vi "User.LoginGui.vi"(11 "Try only (T)":bool=TRUE) -> (2 "UserLevelOut":T1 caption="User Level Out", 3 "ok?":bool)   [LabVIEW 2013]
uses:
  User.LoginGui.Action.ctl
  User.Global.vi
  User.Level.ctl
  Config/Config.Global.vi
panel:
  out "_loop":i32(ring)=4
  in  "open?":bool
  out "_GuruPeriod":string caption="Valid Time"
  in  "SettingsButton":bool
  in  "starthere":dbl
  in  "pwd_Password":string caption="Password"
  out "User":i32(ring) caption="Operator" items=["-", "Guru", "Service", "Operator"]
  in  "CancelButton":bool
  in  "OKButton":bool
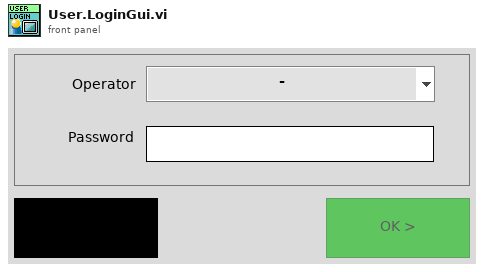
[diagram p1: front panel]
types:
  T1 = typedef "User.Level.ctl" = enum16{"-", "Operator", "Technician", "Administrator"}
  T2 = typedef "User.LoginGui.Action.ctl" = enum32{"idle", "constructor", "destructor", "--- Login GUI ---", "get users"}
  T3 = enum8{"Enabled", "Disabled", "Disabled and Grayed Out"}
  T4 = enum32{"invalid app kind", "Development System", "Run Time System", "Student Edition", "Embedded LabVIEW", "Evaluation", "Custom"}
  T5 = typedef "LVDateTimeRec.ctl" = cluster{"fractional second":dbl, "second":i32, "minute":i32, "hour":i32, "day of month":i32, "month":i32, "year":i32, "day of week":i32, "day of year":i32, "DST":i32}
  T6 = typedef "User.Info.ctl" = cluster{"ID":i32, "Name":string, "Pass":string, "Level":T1, "Del":bool}
  T7 = typedef "LVPositionTypeDef.ctl" = cluster{"Left":i32, "Top":i32}
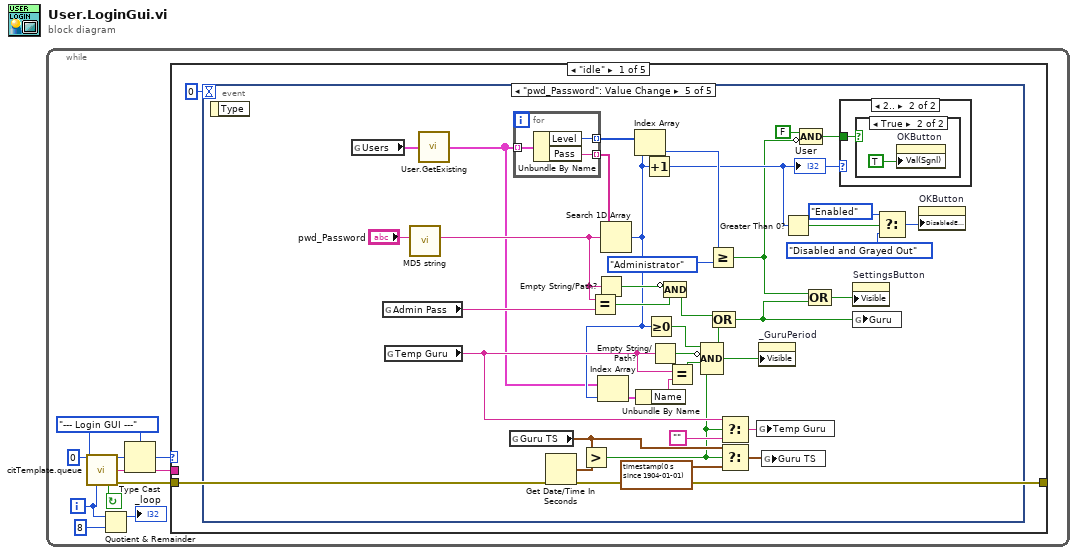
[diagram p0: block diagram]
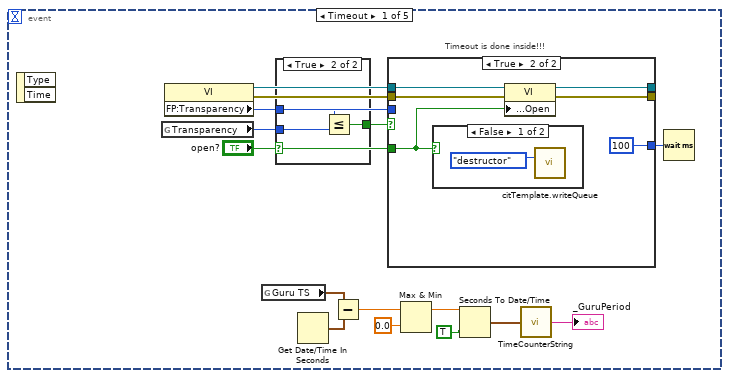
[diagram p2: hidden frame]
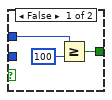
[diagram p3: hidden frame]
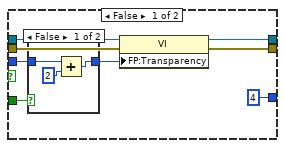
[diagram p4: hidden frame]
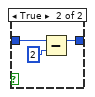
[diagram p5: hidden frame]
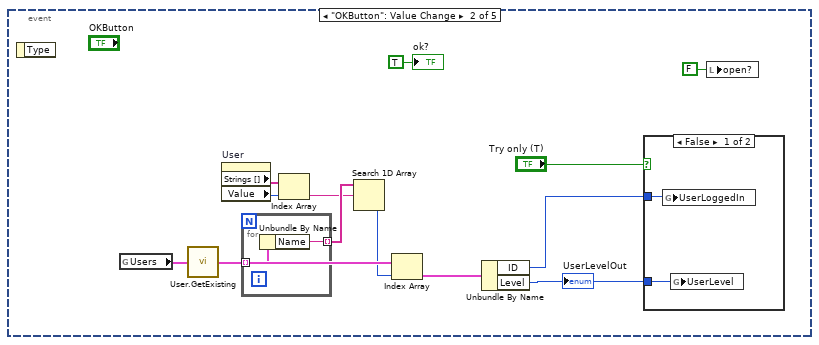
[diagram p7: hidden frame]
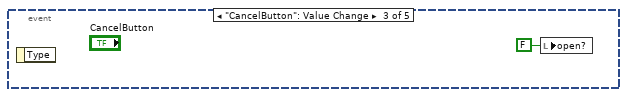
[diagram p9: hidden frame]
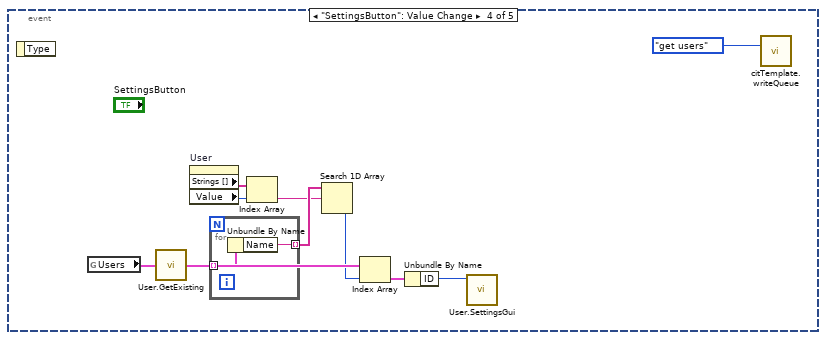
[diagram p10: hidden frame]
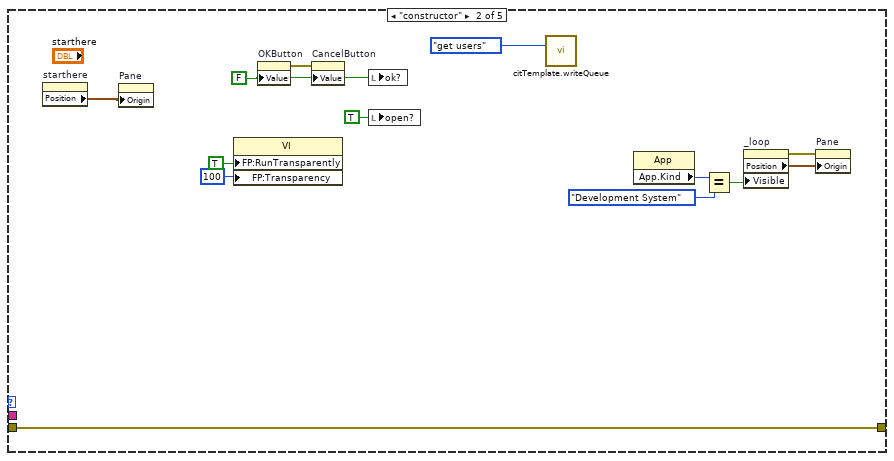
[diagram p13: hidden frame]
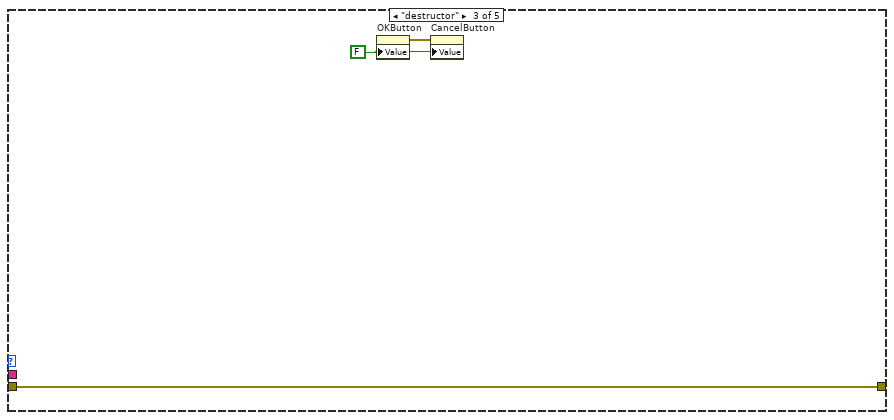
[diagram p14: hidden frame]
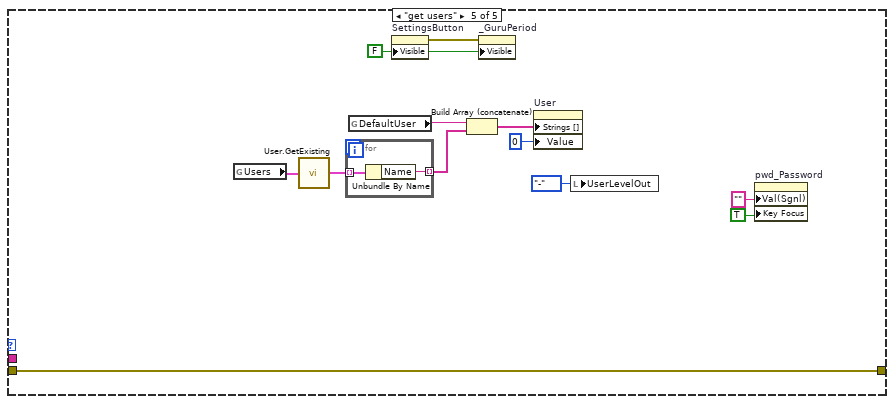
[diagram p16: hidden frame]
diagram:
  n1 = while {
    i -> [w1]
    stop <- w7 continue-if-true
    w6 = User.LoginGui.Action."--- Login GUI ---" ("Action")
    n2 = call "citTemplate.queue.vi"("ms timeout (250 ms)"=0, "event enum"=w6, "iteration (-1)"=w1) -> ("event out"=w10:u32, "(flatten) data out"=w9:string, "continue"=w7:bool, "error out"=w8:errorcluster)  [unwired: 2 in, 7 out]
    n3 = Quotient & Remainder(x=w1, y=8) -> (x-y*floor(x/y)=→"_loop":i32)  [unwired: 1 out]
    n4 = Type Cast(type=w6, x=w10) -> (*(type *) &x=w5:T2)
    n5 = case shown="\"idle\"" w5 {
      tunnel: w9 -> [_ _ _ _ _]
      tunnel: w8 -> [w11 w127 w140 w143 w152]
      tunnel: [w11 w127 w140 w143 w152] -> _
      frame "idle" {
        n6 = event shown="[4] \"pwd_Password\": Value Change" {
          selector: _ -> [_ _ _ _ _]
          dyn-events: _ -> [_ _ _ _ _]
          timeout: 0 -> [_ _ _ _ _]
          event Timeout {
            # "Timeout is done inside!!!"
            n7 = event-data() -> ()  [unwired: 1 in, 2 out]
            n8 = global read "Config.Global.vi" "Transparency"() -> (w14:u8)
            n9 = property class="VI"() -> (reference out=w17:refnum<vi>, error out=w16:errorcluster, "FP:Transparency"=w18:u8)  [unwired: 2 in]
            n10 = global read "User.Global.vi" "Guru TS"() -> (w25:timestamp)
            n11 = case shown="True" "open?" {
              tunnel: w18 -> [w29 w33]
              tunnel: [w28 w32] -> w19
              tunnel: w14 -> [_ w31]
              frame False {
                n12 = Greater Or Equal?(x=w29, y=u8 100) -> (x >= y?=w28:bool)
              }
              frame True {
                n13 = Less Or Equal?(x=w33, y=w31) -> (x <= y?=w32:bool)
              }
            }
            n14 = Get Date/Time In Seconds() -> (seconds since 1Jan1904=w26:timestamp)
            n15 = Subtract(x=w25, y=w26) -> (x-y=w24:dbl)
            n16 = case shown="True" w19 {
              tunnel: w16 -> [w41 w53]
              tunnel: w17 -> [w40 w52]
              tunnel: w18 -> [w39 _]
              tunnel: "open?" -> [w38 w48]
              tunnel: [w36 w51] -> _
              tunnel: [w35 w50] -> _
              tunnel: [u32 4 ("milliseconds to wait") u32 100 ("ms timeout (250 ms)")] -> w13
              frame False {
                n17 = case shown="False" w38 {
                  tunnel: w39 -> [w44 w46]
                  tunnel: [w43 w45] -> w37
                  frame False {
                    n18 = Add(x=w44, y=u8 2 ("x")) -> (x+y=w43:u8)
                  }
                  frame True {
                    n19 = Subtract(x=w46, y=u8 2 ("x")) -> (x-y=w45:u8)
                  }
                }
                n20 = property class="VI"(reference=w40, error in=w41, "FP:Transparency"=w37) -> (reference out=w35:refnum<vi>, error out=w36:errorcluster)
              }
              frame True {
                n21 = case shown="False" w48 {
                  frame False {
                    n22 = call "citTemplate.writeQueue.vi"("event in (if not connected:all statemachine with data event)"=User.LoginGui.Action."destructor" ("Action")) -> ()  [unwired: 4 in, 11 out]
                  }
                  frame True {
                  }
                }
                n23 = property class="VI"(reference=w52, error in=w53, "Front Panel.Open"=w48) -> (reference out=w50:refnum<vi>, error out=w51:errorcluster)
              }
            }
            n24 = Max & Min(x=w24, y=0.0) -> (max(x,y)=w23:dbl)  [unwired: 1 out]
            n25 = Seconds To Date/Time(time stamp (now)=w23, to UTC (F)=TRUE) -> (date time rec=w21:T5)
            n26 = call "TimeCounterString.vi"("date time rec"=w21) -> ("String"=→"_GuruPeriod":string)  [unwired: 1 in]
            n27 = Wait (ms)(milliseconds to wait=w13) -> ()  [unwired: 1 out]
          }
          event "OKButton": Value Change {
            n28 = event-data() -> ()  [unwired: 1 in, 1 out]
            n29 = global read "User.Global.vi" "Users"() -> (w56:T6[])
            n30 = call "User.GetExisting.vi"("Users in"=w56) -> ("Users out"=w60:T6[])
            n31 = property on="User" class="Ring (strict)"() -> ("Strings []"=w64:string[], "Value"=w63:i32)  [unwired: 2 in, 2 out]
            n32 = for {
              tunnel: w60 -> [w69] mode=indexing
              tunnel: [w68] -> w62 mode=indexing
              n33 = Unbundle By Name(w69) -> ("Name"=w68:string)
            }
            n34 = Index Array(array=w64, index=w63) -> (element=w61:string)
            n35 = Search 1D Array(1D array=w62, element=w61) -> (index of element=w59:i32)  [unwired: 1 in]
            n36 = Index Array(array=w60, index=w59) -> (element=w58:T6)
            n37 = Unbundle By Name(w58) -> ("ID"=w57:i32, "Level"=w65:T1)
            "UserLevelOut" <- w65
            n38 = case shown="False" "Try only (T)" {
              tunnel: w65 -> [w71 _]
              tunnel: w57 -> [w70 _]
              frame False {
                n39 = global write "User.Global.vi" "UserLoggedIn"(w70) -> ()
                n40 = global write "User.Global.vi" "UserLevel"(w71) -> ()
              }
              frame True {
              }
            }
            n41 = local write "open?"(FALSE ("open?")) -> ()
            "ok?" <- TRUE ("ok?")
          }
          event "CancelButton": Value Change {
            n42 = event-data() -> ()  [unwired: 1 in, 1 out]
            n43 = local write "open?"(FALSE ("open?")) -> ()
          }
          event "SettingsButton": Value Change {
            n44 = event-data() -> ()  [unwired: 1 in, 1 out]
            n45 = global read "User.Global.vi" "Users"() -> (w74:T6[])
            n46 = call "User.GetExisting.vi"("Users in"=w74) -> ("Users out"=w77:T6[])
            n47 = property on="User" class="Ring (strict)"() -> ("Strings []"=w81:string[], "Value"=w80:i32)  [unwired: 2 in, 2 out]
            n48 = for {
              tunnel: w77 -> [w84] mode=indexing
              tunnel: [w83] -> w79 mode=indexing
              n49 = Unbundle By Name(w84) -> ("Name"=w83:string)
            }
            n50 = Index Array(array=w81, index=w80) -> (element=w78:string)
            n51 = Search 1D Array(1D array=w79, element=w78) -> (index of element=w76:i32)  [unwired: 1 in]
            n52 = Index Array(array=w77, index=w76) -> (element=w75:T6)
            n53 = Unbundle By Name(w75) -> ("ID"=w73:i32)
            n54 = call "User.SettingsGui.vi"("User in"=w73) -> ()  [unwired: 11 in]
            n55 = call "citTemplate.writeQueue.vi"("event in (if not connected:all statemachine with data event)"=User.LoginGui.Action."get users" ("Action")) -> ()  [unwired: 14 in, 1 out]
          }
          event "pwd_Password": Value Change {
            n56 = event-data() -> ()  [unwired: 1 in, 1 out]
            n57 = global read "User.Global.vi" "Users"() -> (w87:T6[])
            n58 = global read "User.Global.vi" "Admin Pass"() -> (w116:string)
            n59 = global read "User.Global.vi" "Temp Guru"() -> (w92:string)
            n60 = call "MD5 string.vi"("Message String"="pwd_Password") -> ("MD5 message-digest"=w96:string)  [unwired: 10 in]
            n61 = call "User.GetExisting.vi"("Users in"=w87) -> ("Users out"=w86:T6[])
            n62 = global read "User.Global.vi" "Guru TS"() -> (w106:timestamp)
            n63 = for {
              tunnel: w86 -> [w124] mode=indexing
              tunnel: [w123] -> w111 mode=indexing
              tunnel: [w122] -> w115 mode=indexing
              n64 = Unbundle By Name(w124) -> ("Level"=w122:T1, "Pass"=w123:string)
            }
            n65 = Get Date/Time In Seconds() -> (seconds since 1Jan1904=w107:timestamp)
            n66 = Greater?(x=w106, y=w107) -> (0:w88:bool)
            n67 = Equal?(x=w96, y=w116) -> (x = y?=w94:bool)
            n68 = Empty String/Path?(string/path=w96) -> (empty?=w95:bool)
            n69 = Search 1D Array(1D array=w111, element=w96) -> (index of element=w91:i32)  [unwired: 1 in]
            n70 = Index Array(array=w86, index=w91) -> (element=w101:T6)
            n71 = Index Array(array=w115, index=w91) -> (element=w114:T1)
            n72 = Unbundle By Name(w101) -> ("Name"=w100:string)
            n73 = Increment(x=w91) -> (x+1=w110:i32)
            "User" <- w110
            n74 = Greater Or Equal To 0?(x=w91) -> (x >= 0?=w98:bool)
            n75 = Empty String/Path?(string/path=w92) -> (empty?=w99:bool)
            n76 = Compound Arithmetic op=AND(invert w95, w94) -> (w93:bool)
            n77 = Equal?(x=w92, y=w100) -> (x = y?=w97:bool)
            n78 = Compound Arithmetic op=AND(w98, invert w99, w97, w88) -> (w89:bool)
            n79 = Greater Or Equal?(x=w114, y=User.Level."Administrator") -> (x >= y?=w108:bool)
            n80 = Compound Arithmetic op=OR(w93, w89) -> (w90:bool)
            n81 = Select(t=w92, s=w88, f="") -> (s? t:f=w103:string)
            n82 = Select(t=w106, s=w88, f=timestamp(0 s since 1904-01-01)) -> (s? t:f=w105:timestamp)
            n83 = global write "User.Global.vi" "Temp Guru"(w103) -> ()
            n84 = property on="_GuruPeriod" class="Str"("Visible"=w89) -> ()  [unwired: 2 in, 2 out]
            n85 = global write "User.Global.vi" "Guru TS"(w105) -> ()
            n86 = Greater Than 0?(x=w110) -> (x > 0?=w117:bool)
            n87 = Compound Arithmetic op=AND(FALSE ("value"), invert w108) -> (w109:bool)
            n88 = Compound Arithmetic op=OR(w108, w90) -> (w112:bool)
            n89 = case shown="2.." w110 {
              tunnel: w109 -> [_ w125]
              frame 0, Default {
              }
              frame 2.. {
                n90 = case shown="True" w125 {
                  frame False {
                  }
                  frame True {
                    n91 = property on="OKButton" class="Bool (strict)"("Val(Sgnl)"=TRUE ("Value (Signaling)")) -> ()  [unwired: 2 in, 2 out]
                  }
                }
              }
            }
            n92 = property on="SettingsButton" class="Bool"("Visible"=w112) -> ()  [unwired: 2 in, 2 out]
            n93 = global write "User.Global.vi" "Guru"(w90) -> ()
            n94 = Select(t=T3."Enabled" ("Disabled"), s=w117, f=T3."Disabled and Grayed Out" ("Disabled")) -> (s? t:f=w120:T3)
            n95 = property on="OKButton" class="Bool (strict)"("DisabledEnum"=w120) -> ()  [unwired: 2 in, 2 out]
          }
        }
      }
      frame "constructor" {
        w136 = FALSE ("_b_OK")
        n96 = property on="starthere" class="DigNum (strict)"() -> ("Position"=w139:T7)  [unwired: 2 in, 2 out]
        n97 = property on="Pane" class="Pane"("Origin"=w139) -> ()  [unwired: 2 in, 2 out]
        n98 = property class="VI"("FP:RunTransparently"=TRUE ("Front Panel Window:Run VI Transparently"), "FP:Transparency"=u8 100 ("Front Panel Window:Transparency")) -> ()  [unwired: 2 in, 2 out]
        n99 = property on="OKButton" class="Bool (strict)"("Value"=w136) -> (error out=w137:errorcluster)  [unwired: 2 in, 1 out]
        n100 = property on="CancelButton" class="Bool (strict)"(error in=w137, "Value"=w136) -> ()  [unwired: 1 in, 2 out]
        n101 = local write "ok?"(w136) -> ()
        n102 = local write "open?"(TRUE ("open?")) -> ()
        n103 = call "citTemplate.writeQueue.vi"("event in (if not connected:all statemachine with data event)"=User.LoginGui.Action."get users" ("Action")) -> ()  [unwired: 14 in, 1 out]
        n104 = property class="App"() -> ("App.Kind"=w130:T4)  [unwired: 2 in, 2 out]
        n105 = Equal?(x=w130, y=T4."Development System") -> (x = y?=w128:bool)
        n106 = property on="_loop" class="Ring (strict)"("Visible"=w128) -> (error out=w132:errorcluster, "Position"=w133:T7)  [unwired: 2 in, 1 out]
        n107 = property on="Pane" class="Pane"(error in=w132, "Origin"=w133) -> ()  [unwired: 1 in, 2 out]
      }
      frame "destructor" {
        w141 = FALSE ("_b_OK")
        n108 = property on="OKButton" class="Bool (strict)"("Value"=w141) -> (error out=w142:errorcluster)  [unwired: 2 in, 1 out]
        n109 = property on="CancelButton" class="Bool (strict)"(error in=w142, "Value"=w141) -> ()  [unwired: 1 in, 2 out]
      }
      frame "--- Login GUI ---" {
      }
      frame "get users" {
        w151 = FALSE ("Visible")
        n110 = global read "User.Global.vi" "Users"() -> (w146:T6[])
        n111 = call "User.GetExisting.vi"("Users in"=w146) -> ("Users out"=w145:T6[])
        n112 = for {
          tunnel: w145 -> [w157] mode=indexing
          tunnel: [w156] -> w144 mode=indexing
          n113 = Unbundle By Name(w157) -> ("Name"=w156:string)
        }
        n114 = global read "User.Global.vi" "DefaultUser"() -> (w153:string)
        n115 = property on="SettingsButton" class="Bool"("Visible"=w151) -> (error out=w150:errorcluster)  [unwired: 2 in, 1 out]
        n116 = Build Array (concatenate)(w153, w144) -> (w155:string[])
        n117 = property on="_GuruPeriod" class="Str"(error in=w150, "Visible"=w151) -> ()  [unwired: 1 in, 2 out]
        n118 = property on="User" class="Ring (strict)"("Strings []"=w155, "Value"=0 ("UserLoggedIn")) -> ()  [unwired: 2 in, 2 out]
        n119 = local write "UserLevelOut"(User.Level."-" ("UserLevelOut")) -> ()
        n120 = property on="pwd_Password" class="Str"("Val(Sgnl)"="" ("Password"), "Key Focus"=TRUE) -> ()  [unwired: 2 in, 2 out]
      }
    }
  }
